vi "TDS Disconnect All.vi"(8 "error in (no error)":errorcluster, 11 "Address":string) -> (0 "error out":errorcluster)   [LabVIEW 2025, in "Interface Functions.lvlib"]
uses:
  Interface Functions.lvlib
panel:
  # "Disconnect All"
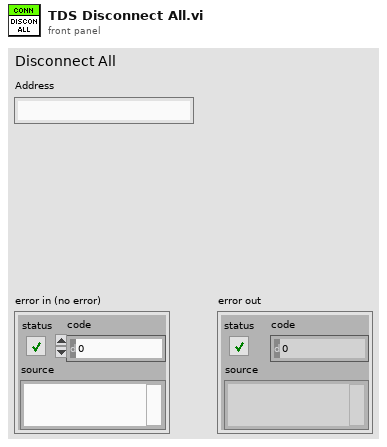
[diagram p1: front panel]
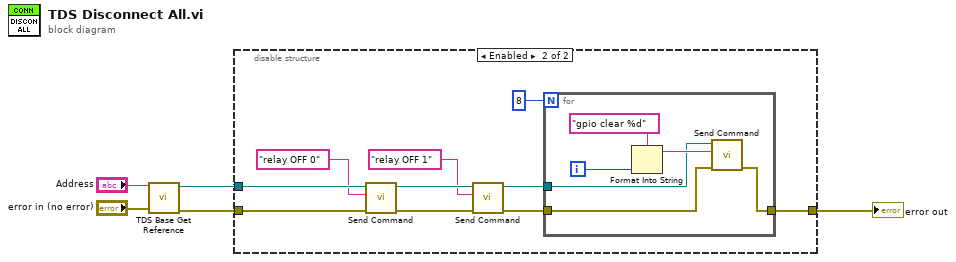
[diagram p0: block diagram]
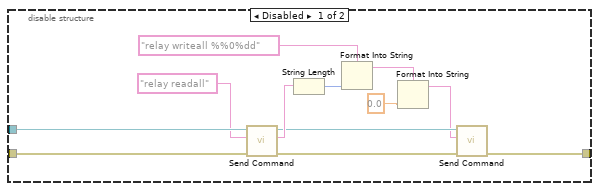
[diagram p2: hidden frame]
diagram:
  n1 = call "TDS Base Get Reference.vi"("error in (no error)"="error in (no error)", "Address"="Address") -> ("error out"=w3:errorcluster, "Reference"=w2:refnum<visa-resource-name>)  [unwired: 8 in]
  n2 = disable-structure shown="Enabled" {
    disable-tunnel: w3 -> [w17 w25]
    disable-tunnel: w2 -> [w16 w27]
    disable-tunnel: [w6 w19] -> w1
    frame Disabled {
      n3 = call "Send Command.vi"("error in (no error)"=w17, "Command"="relay readall", "VISA resource name"=w16) -> ("error out"=w9:errorcluster, "Read Value"=w14:string, "VISA resource name out"=w8:refnum<visa-resource-name>)  [unwired: 6 in]
      n4 = String Length(string=w14) -> (length=w13:i32)
      n5 = Format Into String(format string="relay writeall %%0%dd" ("write buffer"), w13) -> (resulting string=w11:string)  [unwired: 2 in, 1 out]
      n6 = Format Into String(format string=w11, 0.0 ("input 6")) -> (resulting string=w7:string)  [unwired: 2 in, 1 out]
      n7 = call "Send Command.vi"("error in (no error)"=w9, "Command"=w7, "VISA resource name"=w8) -> ("error out"=w6:errorcluster)  [unwired: 6 in, 2 out]
    }
    frame Enabled {
      n8 = call "Send Command.vi"("error in (no error)"=w25, "Command"="relay OFF 0" ("write buffer"), "VISA resource name"=w27) -> ("error out"=w24:errorcluster, "VISA resource name out"=w26:refnum<visa-resource-name>)  [unwired: 6 in, 1 out]
      n9 = call "Send Command.vi"("error in (no error)"=w24, "Command"="relay OFF 1" ("write buffer"), "VISA resource name"=w26) -> ("error out"=w20:errorcluster, "VISA resource name out"=w18:refnum<visa-resource-name>)  [unwired: 6 in, 1 out]
      n10 = for {
        N: 8 -> [_]
        tunnel: w20 -> [w30]
        tunnel: [w29] -> w19
        tunnel: w18 -> [w28]
        i -> [w33]
        n11 = Format Into String(format string="gpio clear %d" ("write buffer"), w33) -> (resulting string=w32:string)  [unwired: 2 in, 1 out]
        n12 = call "Send Command.vi"("error in (no error)"=w30, "Command"=w32, "VISA resource name"=w28) -> ("error out"=w29:errorcluster)  [unwired: 6 in, 2 out]
      }
    }
  }
  "error out" <- w1
